vi "replaceEmptyTagNotation.vi"(8 "error in (no error)":errorcluster, 10 "XML in":string, 11 "ReadElement in":refnum<class "XMLParser.lvclass">) -> (0 "error out":errorcluster, 2 "XML out":string, 3 "ReadElement out":refnum<class "XMLParser.lvclass">)   [LabVIEW 2014, in "XML.lvlib" / "XMLParser.lvclass"]
doc: "This VI searches the XML input and replaces any instances of <emptyTagNotation/> with <emptyTagNotation></emptyTagNotation>"
uses:
  <userlib>/Common/XML/XMLParser/XMLParser.lvclass
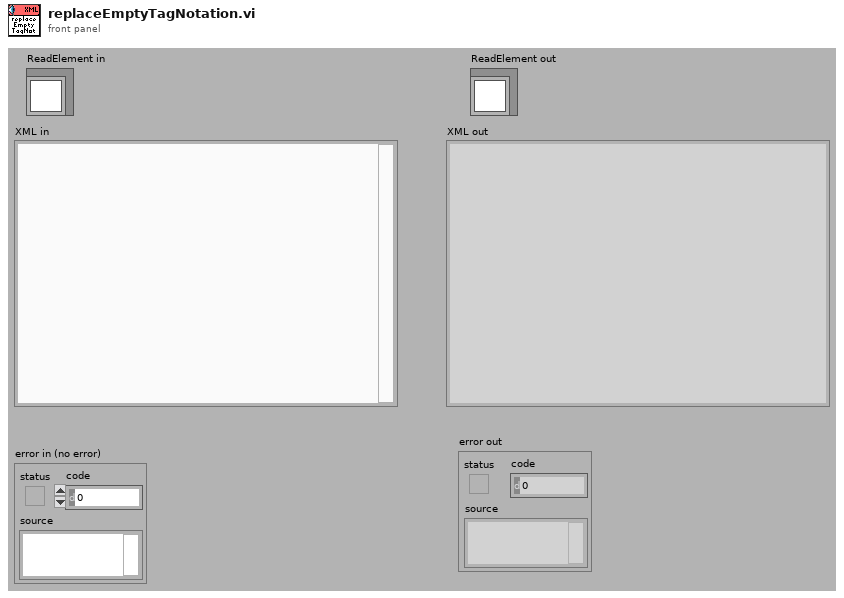
[diagram p1: front panel]
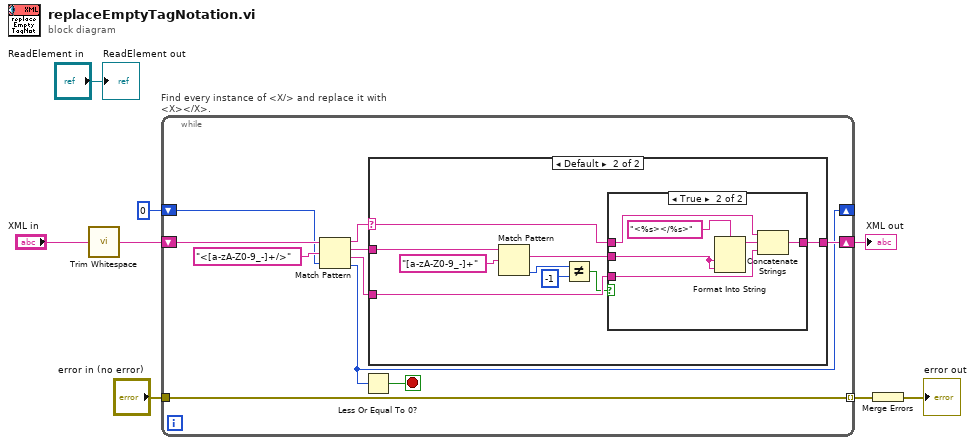
[diagram p0: block diagram]
diagram:
  n1 = call <vilib>:"Trim Whitespace.vi"("string"="XML in") -> ("trimmed string"=w3:string)  [unwired: 1 in]
  n2 = while "Find every instance of <X/> and replace it with <X></X>." {
    shift-right: [w15] -> w4
    shift-left: w3 -> [w17]
    shift-right: [w9] -> _
    shift-left: 0 ("offset (0)") -> [w14]
    tunnel: "error in (no error)" -> [w12]
    tunnel: [w12] -> w5 mode=indexing
    stop <- w13 stop-if-true
    n3 = Match Pattern(string=w17, regular expression="<[a-zA-Z0-9_-]+/>", offset (0)=w14) -> (before substring=w11:string, match substring=w16:string, after substring=w10:string, offset past match=w9:i32)
    n4 = Less Or Equal To 0?(x=w9) -> (x <= 0?=w13:bool)
    n5 = case shown="Default" w11 {
      selector: w11 -> [w19 w23]
      tunnel: w16 -> [_ w28]
      tunnel: w10 -> [_ w26]
      tunnel: [w19 w25] -> w15
      frame "" {
      }
      frame Default {
        n6 = Match Pattern(string=w28, regular expression="[a-zA-Z0-9_-]+") -> (match substring=w24:string, offset past match=w22:i32)  [unwired: 1 in, 2 out]
        n7 = Not Equal?(x=w22, y=-1) -> (x != y?=w20:bool)
        n8 = case shown="True" w20 {
          tunnel: w26 -> [_ w35]
          tunnel: [w29 w34] -> w25
          tunnel: w24 -> [_ w32]
          tunnel: w23 -> [w29 w30]
          frame False {
          }
          frame True {
            n9 = Format Into String(format string="<%s></%s>", w32, w32) -> (resulting string=w31:string)  [unwired: 2 in, 1 out]
            n10 = Concatenate Strings(w30, w31, w35) -> (w34:string)
          }
        }
      }
    }
  }
  "XML out" <- w4
  n11 = Merge Errors(w5) -> (→"error out":errorcluster)
  "ReadElement out" <- "ReadElement in"
